vi "calculate page change.vi"(9 "current page":i32, 10 "set page":i32, 11 "num pages":i32) -> (1 "action":string, 2 "keystroke":string, 3 "page changes rqd":i32)   [LabVIEW 2018]
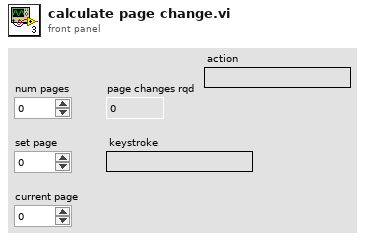
[diagram p1: front panel]
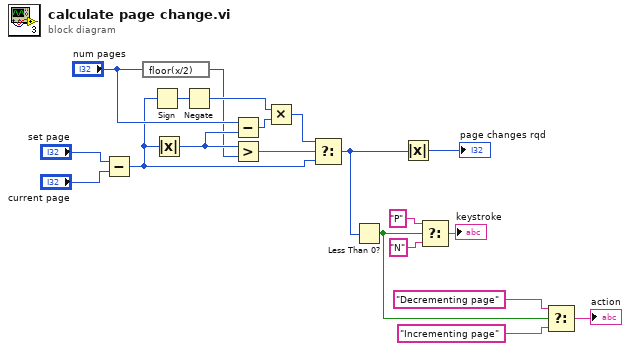
[diagram p0: block diagram]
diagram:
  n1 = Subtract(x="set page", y="current page") -> (x-y=w12:i32)
  n2 = expression code="floor(x/2)"("num pages") -> (w9:i32)
  n3 = Sign(1:w12) -> (0:w14:i32)
  n4 = Absolute Value(x=w12) -> (abs(x)=w10:i32)
  n5 = Negate(x=w14) -> (-x=w13:i32)
  n6 = Subtract(x="num pages", y=w10) -> (x-y=w11:i32)
  n7 = Greater?(x=w10, y=w9) -> (0:w8:bool)
  n8 = Multiply(x=w13, y=w11) -> (x*y=w15:i32)
  n9 = Select(t=w15, s=w8, f=w12) -> (s? t:f=w17:i32)
  n10 = Less Than 0?(x=w17) -> (x < 0?=w2:bool)
  n11 = Absolute Value(x=w17) -> (abs(x)=→"page changes rqd":i32)
  n12 = Select(t="P" ("set Screen"), s=w2, f="N" ("set Screen")) -> (s? t:f=→"keystroke":string)
  n13 = Select(t="Decrementing page" ("set Screen"), s=w2, f="Incrementing page" ("set Screen")) -> (s? t:f=→"action":string)
